vi "configure.vi"(8 "error in (no error)":errorcluster, 11 "LightSourceDL090909Filament in":refnum<class "LightSourceDL090909Filament.lvclass">) -> (0 "error out":errorcluster, 3 "LightSourceDL090909Filament out":refnum<class "LightSourceDL090909Filament.lvclass">)   [LabVIEW 2010, in "LightSourceDL090909Filament.lvclass"]
doc: "The dynamic dispatch version of this VI loads and displays the configuration file associated with the plug-in object. The user modify and save the configuration data."
uses:
  LightSourceDL090909Filament.lvclass
  type_enum.ctl
  LightSourceDL090909Filament.lvclass/LightSourceDL090909Filament.ctl
  common/classes/GenericComponent/GenericComponent/GenericComponent.lvclass
panel:
  in  "type":T1
  out "LSID":string
  out "Configuration":string
  in  "cancel button":bool
  in  "save button":bool
  in  "Serial number":string
  in  "Model":string
  in  "Manufacturer":string
  # "Configure LightSourceDL090909Filament"
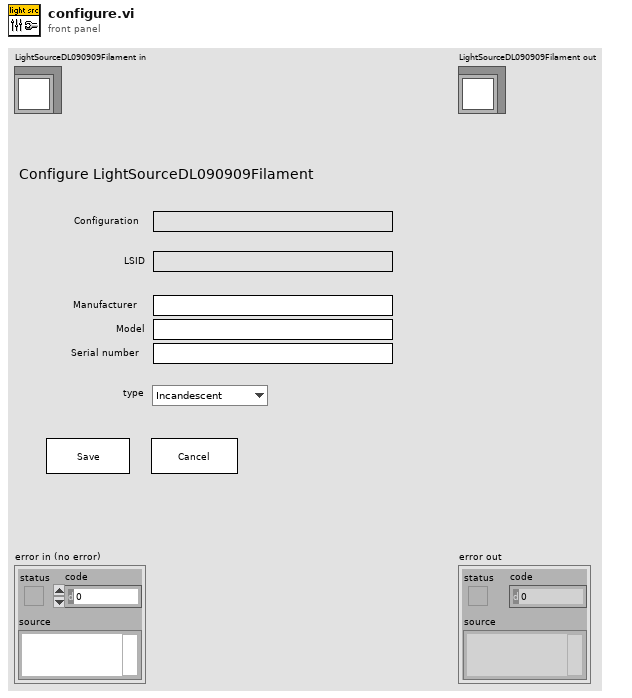
[diagram p1: front panel]
types:
  T1 = typedef "LightSourceDL090909Filament.lvclass/type_enum.ctl" = enum16{"Incandescent", "Halogen", "Unknown"}
  T2 = typedef "LSID_cluster.ctl" = cluster{"identifier":string, "revision":i32}
  T3 = typedef "LightSourceDL090909Filament.lvclass/config_data_cluster.ctl" = cluster{"LSID":T2, "manufacturer specification":T4, "type":T1}
  T4 = typedef "GenericComponent.lvclass/manufacturer_specification_cluster.ctl" = cluster{"manufacturer":string, "model":string, "serial number":string, "lot number":string}
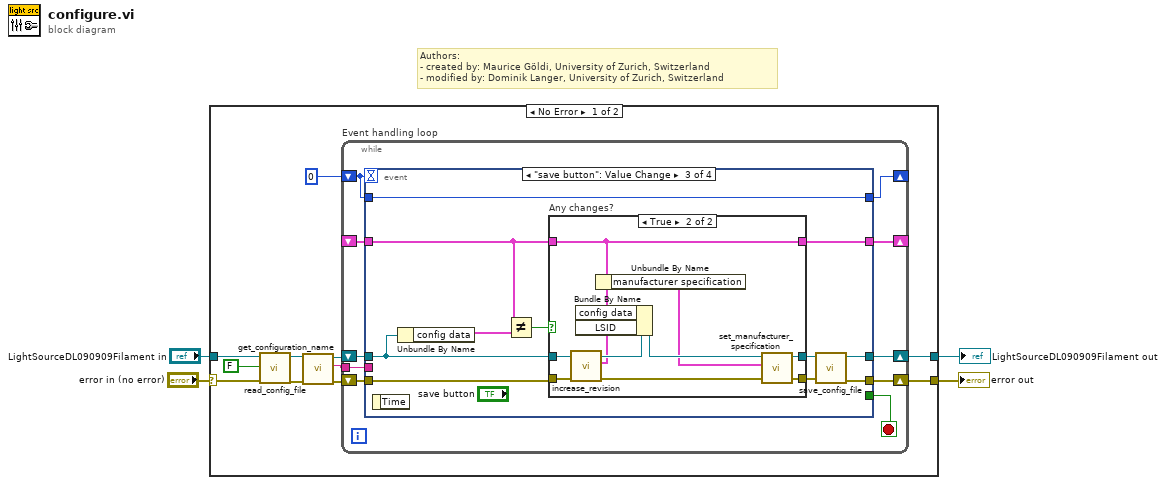
[diagram p0: block diagram]
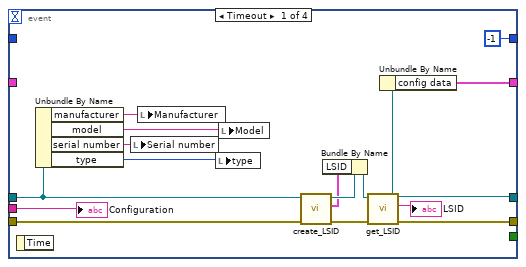
[diagram p2: hidden frame]
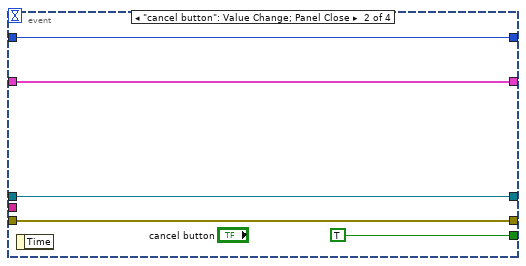
[diagram p3: hidden frame]
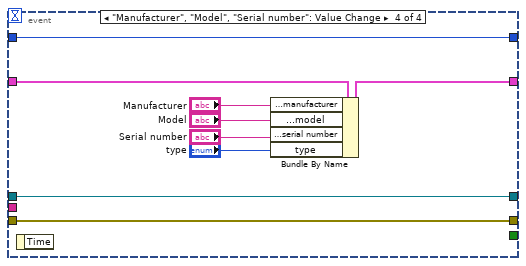
[diagram p5: hidden frame]
diagram:
  # "Authors: \n- created by: Maurice Göldi, University of Zurich, Switzerland\n- modified by: Dominik Langer, University of Zurich, Switzerland"
  n1 = case shown="No Error" "error in (no error)" {
    selector: "error in (no error)" -> [w13 w80]
    tunnel: [w11 w80] -> w4
    tunnel: [w10 w81] -> w3
    tunnel: "LightSourceDL090909Filament in" -> [w14 w81]
    frame No Error {
      n2 = call-dynamic "read_config_file.vi"("error in (no error)"=w13, "force load?"=FALSE, "GenericPlugin in"=w14) -> ("error out"=w8:errorcluster, "GenericPlugin out"=w9:refnum<class "LightSourceDL090909Filament.lvclass">)  [unwired: 7 in]
      n3 = call "get_configuration_name.vi"("error in (no error)"=w8, "GenericPlugin.lvclass in"=w9) -> ("error out"=w7:errorcluster, "configuration name"=w5:string, "GenericPlugin.lvclass out"=w6:refnum<class "LightSourceDL090909Filament.lvclass">)  [unwired: 7 in]
      n4 = while "Event handling loop" {
        shift-right: [w24] -> _
        shift-left: 0 -> [w25]
        shift-right: [w22] -> w11
        shift-left: w7 -> [w23]
        shift-right: [w19] -> w10
        shift-left: w6 -> [w20]
        tunnel: w5 -> [w18]
        shift-right: [w17] -> _
        shift-left: _ -> [w16]
        stop <- w21 stop-if-true
        n5 = event shown="[2] \"save button\": Value Change" {
          selector: _ -> [_ _ _ _]
          dyn-events: _ -> [_ _ _ _]
          timeout: w25 -> [_ _ _ _]
          tunnel: w25 -> [_ w42 w49 w75]
          tunnel: [-1 w42 w49 w75] -> w24
          tunnel: w23 -> [w26 w46 w55 w74]
          tunnel: [w34 w46 w57 w74] -> w22
          tunnel: [_ TRUE _ _] -> w21
          tunnel: w20 -> [w33 w44 w52 w73]
          tunnel: [w28 w44 w53 w73] -> w19
          tunnel: w18 -> [w40 _ _ _]
          tunnel: [w27 w43 w47 w71] -> w17
          tunnel: w16 -> [_ w43 w48 w72]
          event Timeout {
            n6 = event-data() -> ()  [unwired: 1 in, 1 out]
            n7 = Unbundle By Name(w33) -> ("manufacturer"=w39:string, "model"=w38:string, "serial number"=w37:string, "type"=w36:T1)
            n8 = local write "Serial number"(w37) -> ()
            n9 = local write "Manufacturer"(w39) -> ()
            n10 = local write "type"(w36) -> ()
            n11 = local write "Model"(w38) -> ()
            n12 = call-dynamic "create_LSID.vi"("error in (no error)"=w26, "GenericPlugin in"=w33) -> ("error out"=w35:errorcluster, "current LSID"=w31:T2, "GenericPlugin out"=w32:refnum<class "LightSourceDL090909Filament.lvclass">)  [unwired: 7 in]
            n13 = Bundle By Name(cluster=w32, "LSID"=w31) -> (w30:refnum<class "LightSourceDL090909Filament.lvclass">)
            n14 = call-dynamic "get_LSID.vi"("error in (no error)"=w35, "GenericPlugin in"=w30) -> ("error out"=w34:errorcluster, "LSID (string)"=→"LSID":string, "GenericPlugin out"=w28:refnum<class "LightSourceDL090909Filament.lvclass">)  [unwired: 6 in, 1 out]
            n15 = Unbundle By Name(w28) -> ("config data"=w27:T3)
            "Configuration" <- w40
          }
          event "cancel button": Value Change; Panel Close {
            n16 = event-data() -> ()  [unwired: 1 in, 1 out]
          }
          event "save button": Value Change {
            n17 = event-data() -> ()  [unwired: 1 in, 1 out]
            n18 = Unbundle By Name(w52) -> ("config data"=w50:T3)
            n19 = Not Equal?(x=w48, y=w50) -> (x != y?=w51:bool)
            n20 = case "Any changes?" shown="True" w51 {
              tunnel: [w60 w64] -> w56
              tunnel: w55 -> [w60 w70]
              tunnel: w52 -> [w59 w69]
              tunnel: [w59 w62] -> w54
              tunnel: w48 -> [w58 w66]
              tunnel: [w58 w66] -> w47
              frame False {
              }
              frame True {
                n21 = call-dynamic "increase_revision.vi"("error in (no error)"=w70, "GenericPlugin in"=w69) -> ("error out"=w65:errorcluster, "new LSID"=w67:T2, "GenericPlugin out"=w68:refnum<class "LightSourceDL090909Filament.lvclass">)  [unwired: 7 in]
                n22 = Bundle By Name(cluster=w68, "config data"=w66, "LSID"=w67) -> (w63:refnum<class "LightSourceDL090909Filament.lvclass">)
                n23 = Unbundle By Name(w66) -> ("manufacturer specification"=w61:T4)
                n24 = call-dynamic "set_manufacturer_specification.vi"("error in (no error)"=w65, "manufacturer specification"=w61, "GenericPlugin in"=w63) -> ("error out"=w64:errorcluster, "GenericPlugin out"=w62:refnum<class "LightSourceDL090909Filament.lvclass">)  [unwired: 7 in]
              }
            }
            n25 = call-dynamic "save_config_file.vi"("error in (no error)"=w56, "GenericPlugin in"=w54) -> ("error out"=w57:errorcluster, "GenericPlugin out"=w53:refnum<class "LightSourceDL090909Filament.lvclass">)  [unwired: 8 in]
          }
          event "Manufacturer", "Model", "Serial number": Value Change {
            n26 = event-data() -> ()  [unwired: 1 in, 1 out]
            n27 = Bundle By Name(cluster=w72, "manufacturer specification.manufacturer"="Manufacturer", "manufacturer specification.model"="Model", "manufacturer specification.serial number"="Serial number", "type"="type") -> (w71:T3)
          }
        }
      }
    }
    frame Error {
    }
  }
  "error out" <- w4
  "LightSourceDL090909Filament out" <- w3
